vi "Anything to String - backup.vi"(8 "Error In":errorcluster, 9 "Anything":variant, 10 "Read/Write Options":T1, 11 "Format String (%#_13g)":string) -> (0 "Error Out":errorcluster, 1 "Section":string, 2 "Strings[]":string[](array[string]))   [LabVIEW 2020]
doc: "Output a string representation of the specified datatype.\n\nFreeware from Moore Good Ideas, inc: www.MooreGoodIdeas.com. Do not remove this line."
uses:
  <vilib>/Utility/VariantDataType/VariantType.lvlib
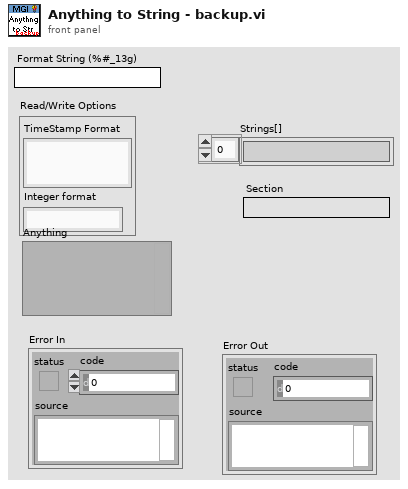
[diagram p1: front panel]
types:
  T1 = cluster{"TimeStamp Format":string, "Integer format":string}
  T2 = typedef "VariantType.lvlib/Type.ctl" = enum8{"Invalid Type", "Void", "I8", "I16", "I32", "I64", "U8", "U16", "U32", "U64", "Single Float", "Double Float", "Extended Float", "Single Complex", "Double Complex", "Extended Complex", "Enum U8", "Enum U16", "Enum U32", "Enum U64", "Single Float With Unit", "Double Float With Unit", "Extended Float With Unit", "Single Complex with Unit", "Double Complex with Unit", "Extended Complex with Unit", "Boolean", "String", "Path", "Picture", "Tag", "Array", "Cluster", "Variant", "LV Variant", "Waveform", "Timestamp", "Digital Waveform", "Digital Data", "ExpressData", "Refnum", "External Data", "VI", "Poly VI", "LabVIEW Class Instance", "Fixed Point"}
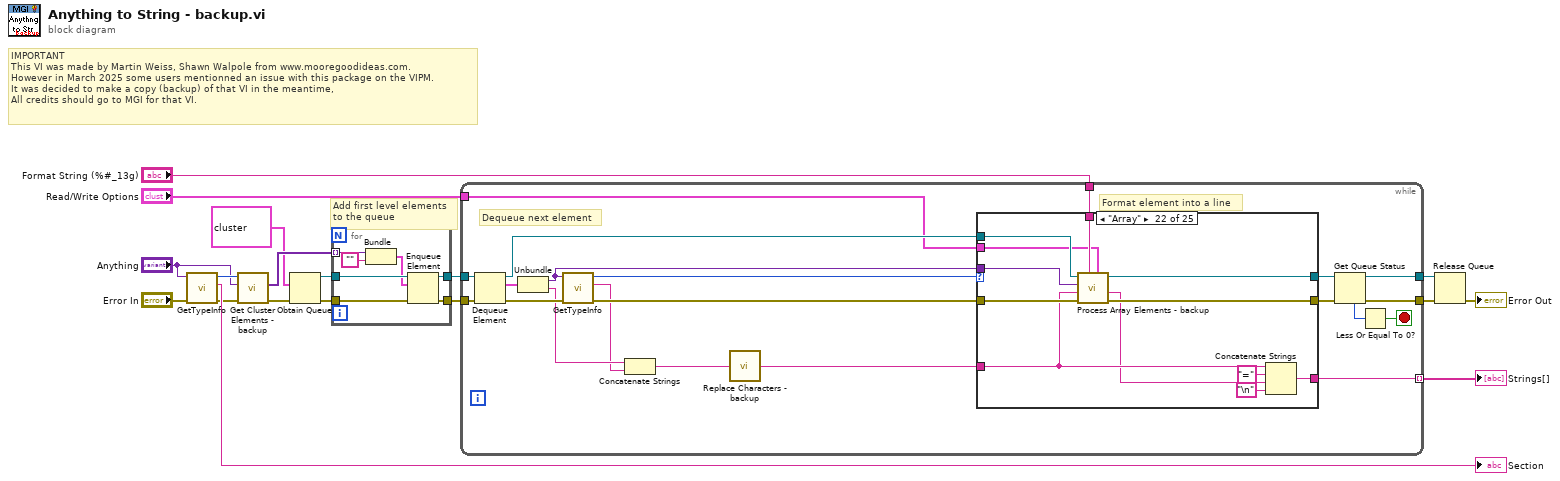
[diagram p0: block diagram]
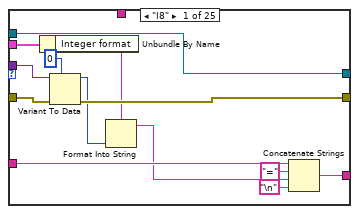
[diagram p2: hidden frame]
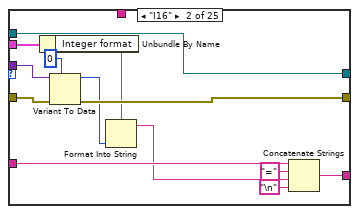
[diagram p3: hidden frame]
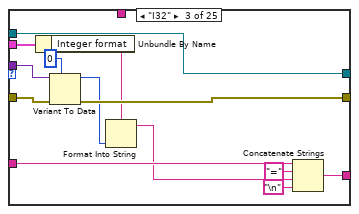
[diagram p4: hidden frame]
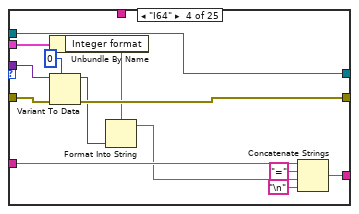
[diagram p5: hidden frame]
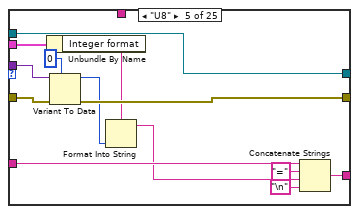
[diagram p6: hidden frame]
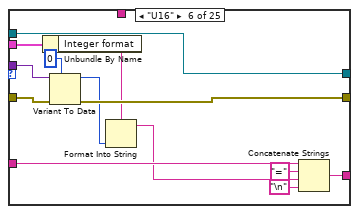
[diagram p7: hidden frame]
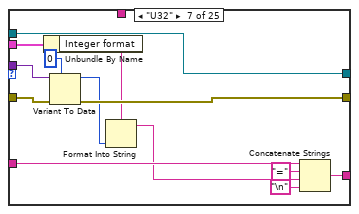
[diagram p8: hidden frame]
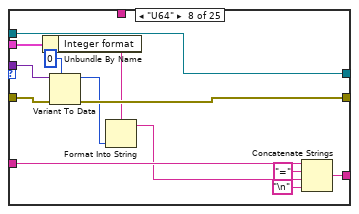
[diagram p9: hidden frame]
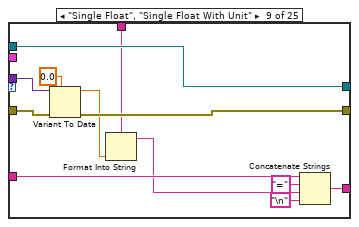
[diagram p10: hidden frame]
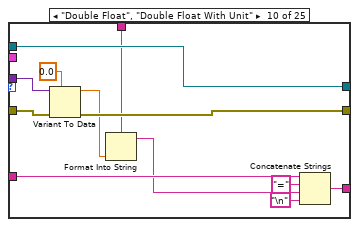
[diagram p11: hidden frame]
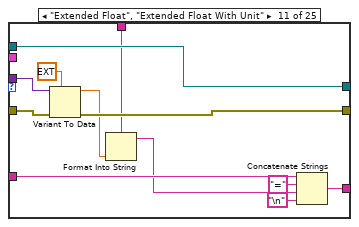
[diagram p12: hidden frame]
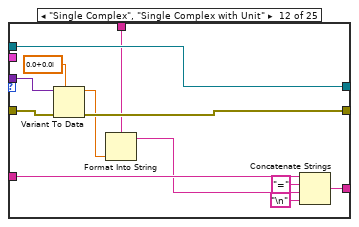
[diagram p13: hidden frame]
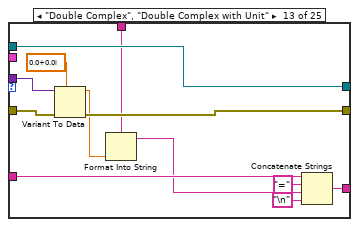
[diagram p14: hidden frame]
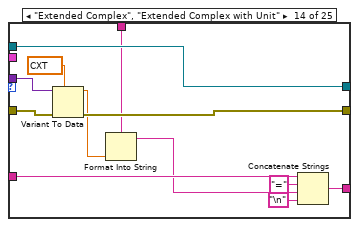
[diagram p15: hidden frame]
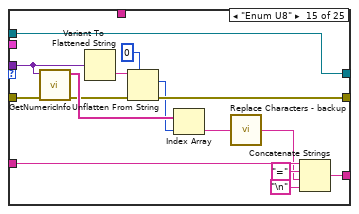
[diagram p16: hidden frame]
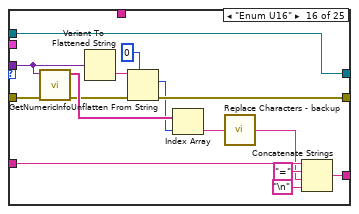
[diagram p17: hidden frame]
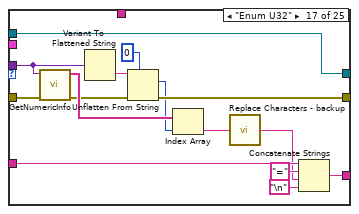
[diagram p18: hidden frame]
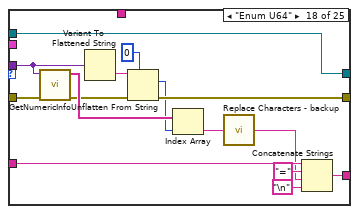
[diagram p19: hidden frame]
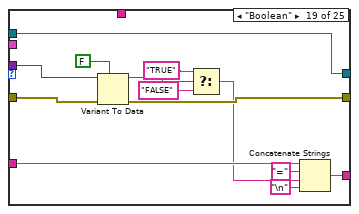
[diagram p20: hidden frame]
diagram:
  # "IMPORTANT\nThis VI was made by Martin Weiss, Shawn Walpole from www.mooregoodideas.com.\nHowever in March 2025 some users mentionned an issue with this package on the VIPM.\nIt was decided to make a copy (backup) of that VI in the meantime,\nAll credits should go to MGI for that VI."
  # "Add first level elements\nto the queue"
  n1 = call <vilib>:"GetTypeInfo.vi"("error in (no error)"="Error In", "Variant"="Anything") -> ("error out"=w9:errorcluster, "Name"=→"Section":string, "Type Enum"=w14:T2)  [unwired: 5 in, 2 out]
  n2 = call "Get Cluster Elements - backup.vi"("Error In"=w9, "Cluster"="Anything", "Type Enum (Cluster)"=w14) -> ("Error Out"=w12:errorcluster, "Cluster Elements"=w11:variant[])  [unwired: 7 in]
  n3 = Obtain Queue(element data type=cluster{"Variant":variant, "Name":string} {"Variant"=variant, "Name"=""}, error in (no error)=w12) -> (queue out=w1:refnum<queue>, error out=w2:errorcluster)  [unwired: 3 in, 1 out]
  n4 = for {
    tunnel: w1 -> [w25]
    tunnel: w2 -> [w24]
    tunnel: [w23] -> w3
    tunnel: [w22] -> w4
    tunnel: w11 -> [w20] mode=indexing
    n5 = Bundle("Variant"=w20, "") -> (w21:cluster{"Variant":variant, string})  [unwired: 1 in]
    n6 = Enqueue Element(queue=w25, element=w21, error in (no error)=w24) -> (queue out=w22:refnum<queue>, error out=w23:errorcluster)  [unwired: 1 in, 1 out]
  }
  n7 = while {
    tunnel: w3 -> [w46]
    tunnel: [w43] -> w5
    tunnel: [w31] -> w18 mode=indexing
    tunnel: w4 -> [w44]
    tunnel: [w40] -> w6
    tunnel: "Format String (%#_13g)" -> [w29]
    tunnel: "Read/Write Options" -> [w28]
    stop <- w41 stop-if-true
    # "Format element into a line"
    # "Dequeue next element"
    n8 = Dequeue Element(queue=w44, error in (no error)=w46) -> (queue out=w37:refnum<queue>, element=w35:cluster{"Variant":variant, "Name":string}, error out=w45:errorcluster)  [unwired: 1 in, 1 out]
    n9 = Unbundle(w35) -> ("Variant"=w34:variant, "Name"=w33:string)
    n10 = call <vilib>:"GetTypeInfo.vi"("error in (no error)"=w45, "Variant"=w34) -> ("error out"=w32:errorcluster, "Name"=w30:string, "Type Enum"=w39:T2)  [unwired: 5 in, 2 out]
    n11 = Concatenate Strings(w33, w30) -> (w27:string)
    n12 = call "Replace Characters - backup.vi"("String In"=w27) -> ("String Out"=w26:string)  [unwired: 1 in]
    n13 = case shown="\"Array\"" w39 {
      selector: w39 -> [_ _ _ _ _ _ _ _ _ _ _ _ _ _ _ _ _ _ _ _ _ _ w336 _ _]
      tunnel: [w59 w72 w85 w98 w111 w124 w137 w150 w162 w174 w186 w198 w210 w222 w237 w252 w267 w282 w295 w306 w318 w326 w340 w362 w370] -> w38
      tunnel: w37 -> [w59 w72 w85 w98 w111 w124 w137 w150 w162 w174 w186 w198 w210 w222 w237 w252 w267 w282 w295 w306 w318 w330 w341 w362 w370]
      tunnel: [w55 w68 w81 w94 w107 w120 w133 w146 w158 w170 w182 w194 w206 w218 w231 w246 w261 w276 w294 w298 w317 w327 w342 w361 w363] -> w36
      tunnel: w32 -> [w58 w71 w84 w97 w110 w123 w136 w149 w161 w173 w185 w197 w209 w221 w236 w251 w266 w281 w291 w301 w314 w328 w338 w361 w364]
      tunnel: w26 -> [w52 w64 w77 w90 w103 w116 w129 w142 w154 w166 w178 w189 w201 w213 w225 w240 w255 w270 w284 w302 w309 w322 w332 w351 w369]
      tunnel: w34 -> [w57 w70 w83 w96 w109 w122 w135 w148 w160 w172 w184 w196 w208 w220 w234 w249 w264 w279 w292 w297 w315 w329 w335 w360 w365]
      tunnel: [w51 w65 w78 w91 w104 w117 w130 w143 w155 w167 w179 w190 w202 w214 w226 w241 w256 w271 w285 w303 w310 w323 _ w352 w371] -> w31
      tunnel: w29 -> [_ _ _ _ _ _ _ _ w151 w164 w175 w187 w199 w211 _ _ _ _ _ _ _ w320 _ _ _]
      tunnel: w28 -> [w48 w61 w74 w87 w100 w113 w126 w139 _ _ _ _ _ _ _ _ _ _ _ _ _ w319 _ _ w367]
      frame "I8" {
        n14 = Unbundle By Name(w48) -> ("Integer format"=w47:string)
        n15 = Variant To Data(error in=w58, type=i8 0, Variant=w57) -> (data=w50:i8, error out=w55:errorcluster)
        n16 = Format Into String(format string=w47, w50) -> (resulting string=w49:string)  [unwired: 2 in, 1 out]
        n17 = Concatenate Strings(w52, "=" ("string"), w49, "\n") -> (w51:string)
      }
      frame "I16" {
        n18 = Unbundle By Name(w61) -> ("Integer format"=w60:string)
        n19 = Variant To Data(error in=w71, type=i16 0, Variant=w70) -> (data=w62:i16, error out=w68:errorcluster)
        n20 = Format Into String(format string=w60, w62) -> (resulting string=w63:string)  [unwired: 2 in, 1 out]
        n21 = Concatenate Strings(w64, "=" ("string"), w63, "\n") -> (w65:string)
      }
      frame "I32" {
        n22 = Unbundle By Name(w74) -> ("Integer format"=w73:string)
        n23 = Variant To Data(error in=w84, type=0, Variant=w83) -> (data=w76:i32, error out=w81:errorcluster)
        n24 = Format Into String(format string=w73, w76) -> (resulting string=w75:string)  [unwired: 2 in, 1 out]
        n25 = Concatenate Strings(w77, "=" ("string"), w75, "\n") -> (w78:string)
      }
      frame "I64" {
        n26 = Unbundle By Name(w87) -> ("Integer format"=w86:string)
        n27 = Variant To Data(error in=w97, type=i64 0, Variant=w96) -> (data=w89:i64, error out=w94:errorcluster)
        n28 = Format Into String(format string=w86, w89) -> (resulting string=w88:string)  [unwired: 2 in, 1 out]
        n29 = Concatenate Strings(w90, "=" ("string"), w88, "\n") -> (w91:string)
      }
      frame "U8" {
        n30 = Unbundle By Name(w100) -> ("Integer format"=w99:string)
        n31 = Variant To Data(error in=w110, type=u8 0, Variant=w109) -> (data=w102:u8, error out=w107:errorcluster)
        n32 = Format Into String(format string=w99, w102) -> (resulting string=w101:string)  [unwired: 2 in, 1 out]
        n33 = Concatenate Strings(w103, "=" ("string"), w101, "\n") -> (w104:string)
      }
      frame "U16" {
        n34 = Unbundle By Name(w113) -> ("Integer format"=w112:string)
        n35 = Variant To Data(error in=w123, type=u16 0, Variant=w122) -> (data=w115:u16, error out=w120:errorcluster)
        n36 = Format Into String(format string=w112, w115) -> (resulting string=w114:string)  [unwired: 2 in, 1 out]
        n37 = Concatenate Strings(w116, "=" ("string"), w114, "\n") -> (w117:string)
      }
      frame "U32" {
        n38 = Unbundle By Name(w126) -> ("Integer format"=w125:string)
        n39 = Variant To Data(error in=w136, type=u32 0, Variant=w135) -> (data=w128:u32, error out=w133:errorcluster)
        n40 = Format Into String(format string=w125, w128) -> (resulting string=w127:string)  [unwired: 2 in, 1 out]
        n41 = Concatenate Strings(w129, "=" ("string"), w127, "\n") -> (w130:string)
      }
      frame "U64" {
        n42 = Unbundle By Name(w139) -> ("Integer format"=w138:string)
        n43 = Variant To Data(error in=w149, type=u64 0, Variant=w148) -> (data=w141:u64, error out=w146:errorcluster)
        n44 = Format Into String(format string=w138, w141) -> (resulting string=w140:string)  [unwired: 2 in, 1 out]
        n45 = Concatenate Strings(w142, "=" ("string"), w140, "\n") -> (w143:string)
      }
      frame "Single Float", "Single Float With Unit" {
        n46 = Variant To Data(error in=w161, type=sgl 0.0, Variant=w160) -> (data=w153:sgl, error out=w158:errorcluster)
        n47 = Format Into String(format string=w151, w153) -> (resulting string=w152:string)  [unwired: 2 in, 1 out]
        n48 = Concatenate Strings(w154, "=" ("string"), w152, "\n") -> (w155:string)
      }
      frame "Double Float", "Double Float With Unit" {
        n49 = Variant To Data(error in=w173, type=0.0, Variant=w172) -> (data=w165:dbl, error out=w170:errorcluster)
        n50 = Format Into String(format string=w164, w165) -> (resulting string=w163:string)  [unwired: 2 in, 1 out]
        n51 = Concatenate Strings(w166, "=" ("string"), w163, "\n") -> (w167:string)
      }
      frame "Extended Float", "Extended Float With Unit" {
        n52 = Variant To Data(error in=w185, type=ext 0.0, Variant=w184) -> (data=w177:ext, error out=w182:errorcluster)
        n53 = Format Into String(format string=w175, w177) -> (resulting string=w176:string)  [unwired: 2 in, 1 out]
        n54 = Concatenate Strings(w178, "=" ("string"), w176, "\n") -> (w179:string)
      }
      frame "Single Complex", "Single Complex with Unit" {
        n55 = Variant To Data(error in=w197, type=csg 0.0+0.0i, Variant=w196) -> (data=w193:csg, error out=w194:errorcluster)
        n56 = Format Into String(format string=w187, w193) -> (resulting string=w188:string)  [unwired: 2 in, 1 out]
        n57 = Concatenate Strings(w189, "=" ("string"), w188, "\n") -> (w190:string)
      }
      frame "Double Complex", "Double Complex with Unit" {
        n58 = Variant To Data(error in=w209, type=cdb 0.0+0.0i, Variant=w208) -> (data=w205:cdb, error out=w206:errorcluster)
        n59 = Format Into String(format string=w199, w205) -> (resulting string=w200:string)  [unwired: 2 in, 1 out]
        n60 = Concatenate Strings(w201, "=" ("string"), w200, "\n") -> (w202:string)
      }
      frame "Extended Complex", "Extended Complex with Unit" {
        n61 = Variant To Data(error in=w221, type=cxt 0.0+0.0i, Variant=w220) -> (data=w217:cxt, error out=w218:errorcluster)
        n62 = Format Into String(format string=w211, w217) -> (resulting string=w212:string)  [unwired: 2 in, 1 out]
        n63 = Concatenate Strings(w213, "=" ("string"), w212, "\n") -> (w214:string)
      }
      frame "Enum U8" {
        n64 = call <vilib>:"GetNumericInfo.vi"("error in (no error)"=w236, "Variant"=w234) -> ("error out"=w232:errorcluster, "EnumNames"=w235:string[])  [unwired: 6 in, 2 out]
        n65 = Variant To Flattened String(Variant=w234) -> (data string=w233:string)  [unwired: 1 out]
        n66 = Unflatten From String(type=u8 0, binary string=w233, error in (no error)=w232) -> (value=w230:u8, error out=w231:errorcluster)  [unwired: 2 in, 1 out]
        n67 = Index Array(array=w235, index=w230) -> (element=w224:string)
        n68 = call "Replace Characters - backup.vi"("String In"=w224) -> ("String Out"=w223:string)  [unwired: 1 in]
        n69 = Concatenate Strings(w225, "=" ("string"), w223, "\n") -> (w226:string)
      }
      frame "Enum U16" {
        n70 = call <vilib>:"GetNumericInfo.vi"("error in (no error)"=w251, "Variant"=w249) -> ("error out"=w247:errorcluster, "EnumNames"=w250:string[])  [unwired: 6 in, 2 out]
        n71 = Variant To Flattened String(Variant=w249) -> (data string=w248:string)  [unwired: 1 out]
        n72 = Unflatten From String(type=u16 0, binary string=w248, error in (no error)=w247) -> (value=w245:u16, error out=w246:errorcluster)  [unwired: 2 in, 1 out]
        n73 = Index Array(array=w250, index=w245) -> (element=w239:string)
        n74 = call "Replace Characters - backup.vi"("String In"=w239) -> ("String Out"=w238:string)  [unwired: 1 in]
        n75 = Concatenate Strings(w240, "=" ("string"), w238, "\n") -> (w241:string)
      }
      frame "Enum U32" {
        n76 = call <vilib>:"GetNumericInfo.vi"("error in (no error)"=w266, "Variant"=w264) -> ("error out"=w262:errorcluster, "EnumNames"=w265:string[])  [unwired: 6 in, 2 out]
        n77 = Variant To Flattened String(Variant=w264) -> (data string=w263:string)  [unwired: 1 out]
        n78 = Unflatten From String(type=u32 0, binary string=w263, error in (no error)=w262) -> (value=w260:u32, error out=w261:errorcluster)  [unwired: 2 in, 1 out]
        n79 = Index Array(array=w265, index=w260) -> (element=w254:string)
        n80 = call "Replace Characters - backup.vi"("String In"=w254) -> ("String Out"=w253:string)  [unwired: 1 in]
        n81 = Concatenate Strings(w255, "=" ("string"), w253, "\n") -> (w256:string)
      }
      frame "Enum U64" {
        n82 = call <vilib>:"GetNumericInfo.vi"("error in (no error)"=w281, "Variant"=w279) -> ("error out"=w277:errorcluster, "EnumNames"=w280:string[])  [unwired: 6 in, 2 out]
        n83 = Variant To Flattened String(Variant=w279) -> (data string=w278:string)  [unwired: 1 out]
        n84 = Unflatten From String(type=u64 0, binary string=w278, error in (no error)=w277) -> (value=w275:u64, error out=w276:errorcluster)  [unwired: 2 in, 1 out]
        n85 = Index Array(array=w280, index=w275) -> (element=w269:string)
        n86 = call "Replace Characters - backup.vi"("String In"=w269) -> ("String Out"=w268:string)  [unwired: 1 in]
        n87 = Concatenate Strings(w270, "=" ("string"), w268, "\n") -> (w271:string)
      }
      frame "Boolean" {
        n88 = Variant To Data(error in=w291, type=FALSE, Variant=w292) -> (data=w290:bool, error out=w294:errorcluster)
        n89 = Select(t="TRUE", s=w290, f="FALSE") -> (s? t:f=w283:string)
        n90 = Concatenate Strings(w284, "=" ("string"), w283, "\n") -> (w285:string)
      }
      frame "String" {
        n91 = Variant To Data(error in=w301, type="", Variant=w297) -> (data=w300:string, error out=w298:errorcluster)
        n92 = call "Replace Characters - backup.vi"("String In"=w300) -> ("String Out"=w299:string)  [unwired: 1 in]
        n93 = Concatenate Strings(w302, "=" ("string"), w299, "\n") -> (w303:string)
      }
      frame "Path" {
        n94 = Variant To Data(error in=w314, type=path "", Variant=w315) -> (data=w313:path, error out=w317:errorcluster)
        n95 = Path To String(path=w313) -> (string=w308:string)
        n96 = call "Replace Characters - backup.vi"("String In"=w308) -> ("String Out"=w307:string)  [unwired: 1 in]
        n97 = Concatenate Strings(w309, "=" ("string"), w307, "\n") -> (w310:string)
      }
      frame "Array" {
        n98 = call "Process Array Elements - backup.vi"("Read/Write Options"=w319, "Format String (%#0.15f)"=w320, "Error In"=w328, "Name In"=w322, "Array Variant"=w329, "Queue In"=w330) -> ("Error Out"=w327:errorcluster, "Data Out"=w321:string, "Queue Out"=w326:refnum<queue>)  [unwired: 3 in]
        n99 = Concatenate Strings(w322, "=" ("string"), w321, "\n") -> (w323:string)
      }
      frame "Cluster" {
        # "Enqueue cluster elements"
        n100 = call "Get Cluster Elements - backup.vi"("Error In"=w338, "Cluster"=w335, "Type Enum (Cluster)"=w336) -> ("Error Out"=w337:errorcluster, "Cluster Elements"=w334:variant[])  [unwired: 7 in]
        n101 = Concatenate Strings(w332, "." ("string")) -> (w331:string)
        n102 = Reverse 1D Array(array=w334) -> (reversed array=w339:variant[])
        n103 = for {
          tunnel: w341 -> [w349]
          tunnel: w337 -> [w348]
          tunnel: [w347] -> w342
          tunnel: [w346] -> w340
          tunnel: w339 -> [w344] mode=indexing
          tunnel: w331 -> [w343]
          n104 = Bundle("Variant"=w344, w343) -> (w345:cluster{"Variant":variant, string})  [unwired: 1 in]
          n105 = Enqueue Element At Opposite End(queue=w349, element=w345, error in (no error)=w348) -> (queue out=w346:refnum<queue>, error out=w347:errorcluster)  [unwired: 1 in, 1 out]
        }
      }
      frame Default {
        n106 = Variant To Flattened String(Variant=w360) -> (data string=w355:string)  [unwired: 1 out]
        n107 = String To Byte Array(string=w355) -> (unsigned byte array=w359:u8[])
        n108 = Number To Hexadecimal String(1:i16 2 ("width (-)"), 2:w359) -> (0:w358:string[])
        n109 = Concatenate Strings("0x", w358) -> (w350:string)
        n110 = Concatenate Strings(w351, "=" ("string"), w350, "\n") -> (w352:string)
      }
      frame "Timestamp" {
        n111 = Unbundle By Name(w367) -> ("TimeStamp Format"=w366:string)
        n112 = case shown="Default" w366 {
          selector: w366 -> [_ w387]
          tunnel: [w377 w388] -> w368
          tunnel: w365 -> [w376 w385]
          tunnel: w364 -> [w374 w384]
          tunnel: [w374 w382] -> w363
          frame "" {
            n113 = Variant To Flattened String(Variant=w376) -> (data string=w375:string)  [unwired: 1 out]
            n114 = String To Byte Array(string=w375) -> (unsigned byte array=w380:u8[])
            n115 = Number To Hexadecimal String(1:i16 2 ("width (-)"), 2:w380) -> (0:w379:string[])
            n116 = Concatenate Strings("0x", w379) -> (w377:string)
          }
          frame Default {
            n117 = Variant To Data(error in=w384, type=timestamp(0 s since 1904-01-01), Variant=w385) -> (data=w383:timestamp, error out=w382:errorcluster)
            n118 = Format Date/Time String(time format string (%c)=w387, seconds (now)=w383) -> (date/time string=w388:string)  [unwired: 1 in]
          }
        }
        n119 = Concatenate Strings(w369, "=" ("string"), w368, "\n") -> (w371:string)
      }
    }
    n120 = Get Queue Status(queue=w38, error in (no error)=w36) -> (queue out=w40:refnum<queue>, error out=w43:errorcluster, # elements in queue=w42:i32)  [unwired: 1 in, 5 out]
    n121 = Less Or Equal To 0?(x=w42) -> (x <= 0?=w41:bool)
  }
  "Strings[]" <- w18
  n122 = Release Queue(queue=w6, error in (no error)=w5) -> (error out=→"Error Out":errorcluster)  [unwired: 1 in, 2 out]
